vi "Exchange Connection Names.vi"(8 "error in (no error)":errorcluster, 10 "Client Name in":string, 11 "connection ID":refnum<k5>) -> (0 "error out":errorcluster, 2 "Server Name out":string, 3 "connection out":refnum<k5>)   [LabVIEW 2017, in "_TCP Client.lvlib" / "TCP Client.lvclass"]
uses:
  TCP Client.lvclass
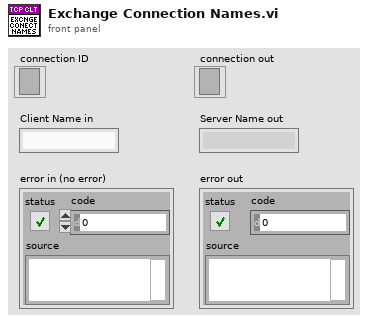
[diagram p1: front panel]
types:
  T1 = enum16{"Standard", "Buffered", "CRLF", "Immediate"}
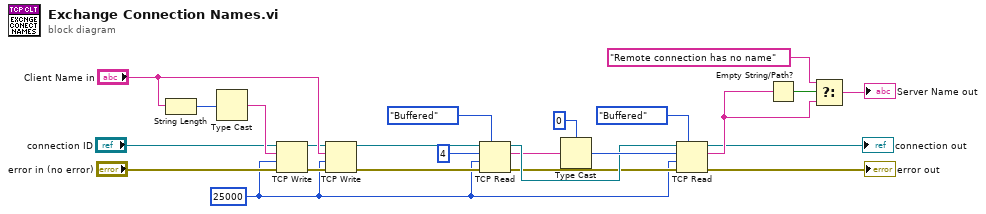
[diagram p0: block diagram]
diagram:
  w1 = 25000 ("timeout ms (25000)")
  n1 = String Length(string="Client Name in") -> (length=w23:i32)
  n2 = Type Cast(x=w23) -> (*(type *) &x=w22:string)  [unwired: 1 in]
  n3 = TCP Write(connection ID="connection ID", data in=w22, error in (no error)="error in (no error)", 9:w1) -> (connection ID out=w20:refnum<k5>, error out=w21:errorcluster)  [unwired: 1 out]
  n4 = TCP Write(connection ID=w20, data in="Client Name in", error in (no error)=w21, 9:w1) -> (connection ID out=w7:refnum<k5>, error out=w3:errorcluster)  [unwired: 1 out]
  n5 = TCP Read(connection ID=w7, bytes to read=4, error in (no error)=w3, 7:T1."Buffered" ("mode (standard)"), 9:w1) -> (connection ID out=w12:refnum<k5>, data out=w11:string, error out=w9:errorcluster)
  n6 = Type Cast(type=0 ("bytes to read"), x=w11) -> (*(type *) &x=w15:i32)
  n7 = TCP Read(connection ID=w12, bytes to read=w15, error in (no error)=w9, 7:T1."Buffered" ("mode (standard)"), 9:w1) -> (connection ID out=→"connection out":refnum<k5>, data out=w18:string, error out=→"error out":errorcluster)
  n8 = Empty String/Path?(string/path=w18) -> (empty?=w16:bool)
  n9 = Select(t="Remote connection has no name", s=w16, f=w18) -> (s? t:f=→"Server Name out":string)
